vi "TC560-Initialize.vi"(8 "error in":errorcluster) -> (0 "error out":errorcluster, 3 "VISA Resource Name":refnum<visa-resource-name>)   [LabVIEW 2018]
uses:
  Data Def/TC560-File Method.ctl
  <vilib>/Instr/_visa.llb/VISA Configure Serial Port (Instr).vi
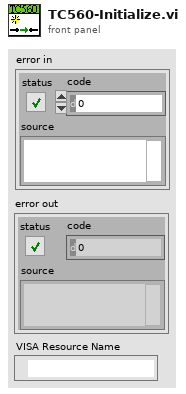
[diagram p1: front panel]
types:
  T1 = typedef "TC560-File Method.ctl" = enum16{"Get", "Put", "Load", "Save"}
  T2 = typedef "TC560-Configuration.ctl" = cluster{"Connection Setting":T3, "Wait For Read":u32}
  T3 = typedef "TC560-Connection Setting.ctl" = cluster{"VISA Resource Name":refnum<visa-resource-name>, "Baud Rate":u32, "Parity":u16, "Flow Control":u16}
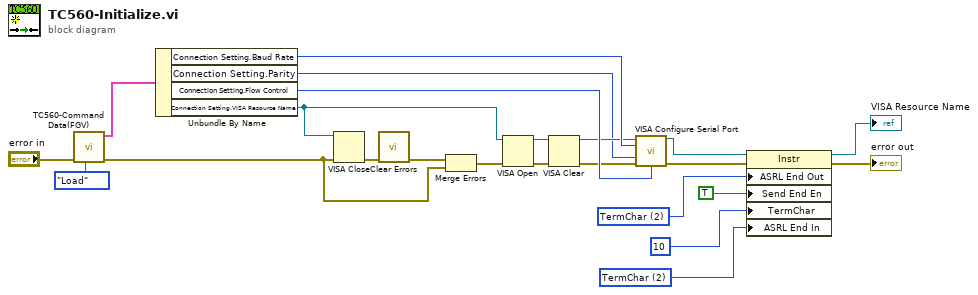
[diagram p0: block diagram]
diagram:
  w8 = u16 2 items=["None", "Last Bit", "TermChar", "Break"] ("Serial Settings:End Mode for Writes")
  w11 = u16 2 items=["None", "Last Bit", "TermChar", "Break"] ("Serial Settings:End Mode for Writes")
  n1 = call "TC560-Command Data(FGV).vi"("File Method"=TC560-File_Method."Load", "error in"="error in") -> ("error out"=w5:errorcluster, "Configuration Out"=w23:T2)  [unwired: 8 in]
  n2 = Unbundle By Name(w23) -> ("Connection Setting.Baud Rate"=w21:u32, "Connection Setting.Parity"=w2:u16, "Connection Setting.Flow Control"=w20:u16, "Connection Setting.VISA Resource Name"=w6:refnum<visa-resource-name>)
  n3 = VISA Close(VISA resource name=w6, error in (no error)=w5) -> (error out=w19:errorcluster)
  n4 = call <vilib>:"Clear Errors.vi"("error in (no error)"=w19) -> ("error out"=w18:errorcluster)  [unwired: 5 in, 1 out]
  n5 = Merge Errors(w18, w5) -> (w7:errorcluster)
  n6 = VISA Open(error in (no error)=w7, VISA resource name=w6) -> (VISA resource name=w16:refnum<visa-resource-name>, error out=w17:errorcluster)  [unwired: 3 in]
  n7 = VISA Clear(VISA resource name=w16, error in (no error)=w17) -> (VISA resource name out=w14:refnum<visa-resource-name>, error out=w15:errorcluster)
  n8 = call-poly "VISA Configure Serial Port"("VISA resource name"=w14, "baud rate (9600)"=w21, "parity (0:none)"=w2, "error in (no error)"=w15, "flow control (0:none)"=w20) -> ("VISA resource name out"=w12:refnum<visa-resource-name>, "error out"=w13:errorcluster)  [unwired: 9 in]
  n9 = property class="Instr"(reference=w12, error in=w13, "ASRL End Out"=w11, "Send End En"=TRUE ("Message Based Settings:Send End Enable"), "TermChar"=u8 10 ("Message Based Settings:Termination Character"), "ASRL End In"=w8) -> (reference out=→"VISA Resource Name":refnum<visa-resource-name>, error out=→"error out":errorcluster)
